vi "boolean to on off string.vi"(11 "Boolean":bool) -> (2 "Stat Array":string[](array[string]), 3 "Stat":string)   [LabVIEW 2017]
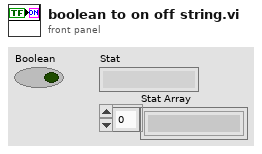
[diagram p1: front panel]
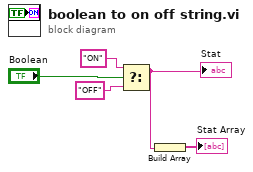
[diagram p0: block diagram]
diagram:
  n1 = Select(t="ON" ("element"), s="Boolean", f="OFF" ("element")) -> (s? t:f=w2:string)
  "Stat" <- w2
  n2 = Build Array(w2) -> (→"Stat Array":string[])
